vi "Var_señales_G1.vi"() -> ()   [LabVIEW 2018]
panel:
  in  "Var_V_G1":sgl
  in  "Var_Frec_G1":sgl
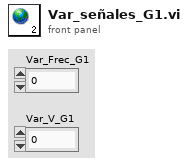
[diagram p1: front panel]
diagram:
